vi "ge_EditPullDown.vi"(4 "CellSize":T2, 6 "ActiveCellPos":T1, 7 "String and Values":cluster{"String":string, "Value":u16}[](array[cluster]), 8 "error in":errorcluster, 10 "PD HiLite":bool, 11 "FP Ctrl":T3) -> (0 "error out":errorcluster, 1 "Discard?":bool)   [LabVIEW 2018]
uses:
  Custom Ctrls/ge_FPCtrlRefLabel.ctl
  <vilib>/Utility/miscctls.llb/LVBoundsTypeDef.ctl
  <vilib>/Utility/miscctls.llb/LVPositionTypeDef.ctl
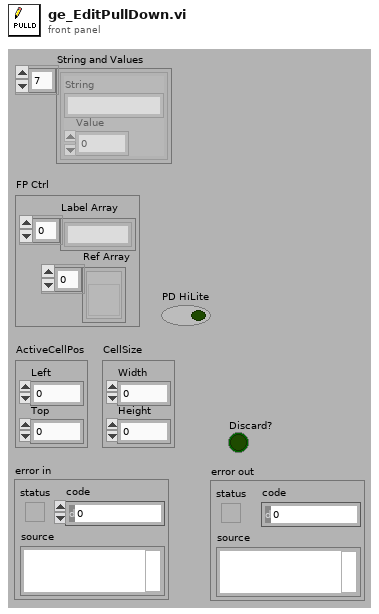
[diagram p1: front panel]
types:
  T1 = typedef "LVPositionTypeDef.ctl" = cluster{"Left":i32, "Top":i32}
  T2 = typedef "LVBoundsTypeDef.ctl" = cluster{"Width":u32, "Height":u32}
  T3 = typedef "ge_FPCtrlRefLabel.ctl" = cluster{"Label Array":string[], "Ref Array":refnum<vi>[]}
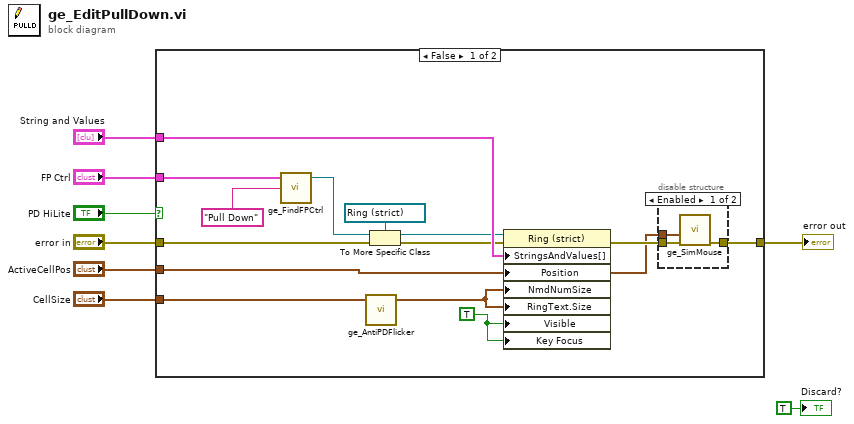
[diagram p0: block diagram]
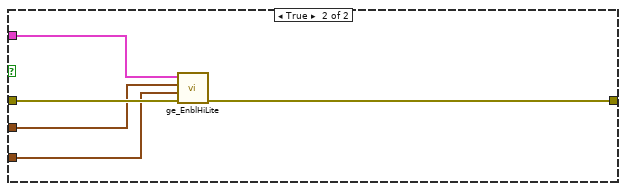
[diagram p3: hidden frame]
diagram:
  n1 = case shown="False" "PD HiLite" {
    tunnel: "CellSize" -> [w22 w28]
    tunnel: "error in" -> [w12 w31]
    tunnel: "ActiveCellPos" -> [w9 w29]
    tunnel: "String and Values" -> [w21 _]
    tunnel: "FP Ctrl" -> [w20 w27]
    tunnel: [w10 w30] -> w3
    frame False {
      w19 = TRUE
      n2 = call "ge_FindFPCtrl.vi"("Ctrl Name"="Pull Down" ("Name"), "FP Ctrl"=w20) -> ("Ctrl Ref"=w15:refnum<vi>)  [unwired: 3 in]
      n3 = call "ge_AntiPDFlicker.vi"("CellSize"=w22) -> ("CellSize"=w14:T2)  [unwired: 4 in]
      n4 = To More Specific Class(target class=refnum<vi> refnum ("reference"), reference=w15, error in=w12) -> (specific class reference=w16:refnum<vi>, error out=w18:errorcluster)
      n5 = property on="Property Node" class="Ring (strict)"(reference=w16, error in=w18, "StringsAndValues[]"=w21, "Position"=w9, "NmdNumSize"=w14, "RingText.Size"=w14, "Visible"=w19, "Key Focus"=w19) -> (error out=w11:errorcluster)  [unwired: 1 out]
      n6 = disable-structure shown="Enabled" {
        disable-tunnel: w11 -> [w25 w26]
        disable-tunnel: [w24 w26] -> w10
        disable-tunnel: w9 -> [w23 _]
        frame Enabled {
          n7 = call "ge_SimMouse.vi"("error in"=w25, "CtrlPos"=w23) -> ("error out"=w24:errorcluster)  [unwired: 8 in]
        }
        frame Disabled {
        }
      }
    }
    frame True {
      n8 = call "ge_EnblHiLite.vi"("error in"=w31, "CellSize"=w28, "ActiveCellPos"=w29, "FP Ctrl"=w27) -> ("error out"=w30:errorcluster)  [unwired: 6 in, 1 out]
    }
  }
  "error out" <- w3
  "Discard?" <- TRUE ("Discard?")
